vi "Read Matlab Params.vi"(8 "error in (no error)":errorcluster, 10 "Enum":T1(ring), 11 "TrialBasedExperiment in":refnum<class "MatlabExperiment.lvclass">) -> (0 "error out":errorcluster, 2 "Matlab Param Array":cluster{"Name":string, "Data":variant}[](array[cluster]), 3 "TrialBasedExperiment out":refnum<class "MatlabExperiment.lvclass">)   [LabVIEW 2010, in "MatlabExperiment.lvclass"]
uses:
  MatlabExperiment.lvclass
  Matlab API/Matlab API.lvlib
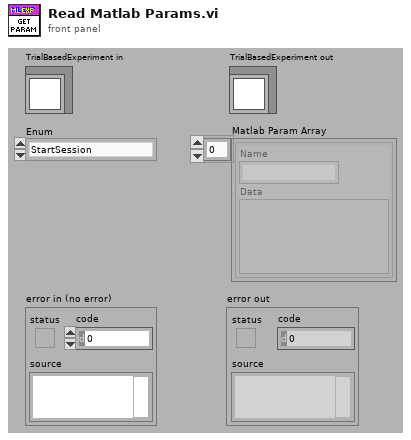
[diagram p1: front panel]
types:
  T1 = enum16{"StartSession", "StartTrial", "ShowStimulus"}
  T2 = cluster{"Name":string, "Type":string, "value":string}[]
  T3 = cluster{"Intertrial":dbl, "AcquireFixation":dbl, "HoldFixation":dbl, "DelayPeriod":dbl, "ResponsePeriod":dbl}
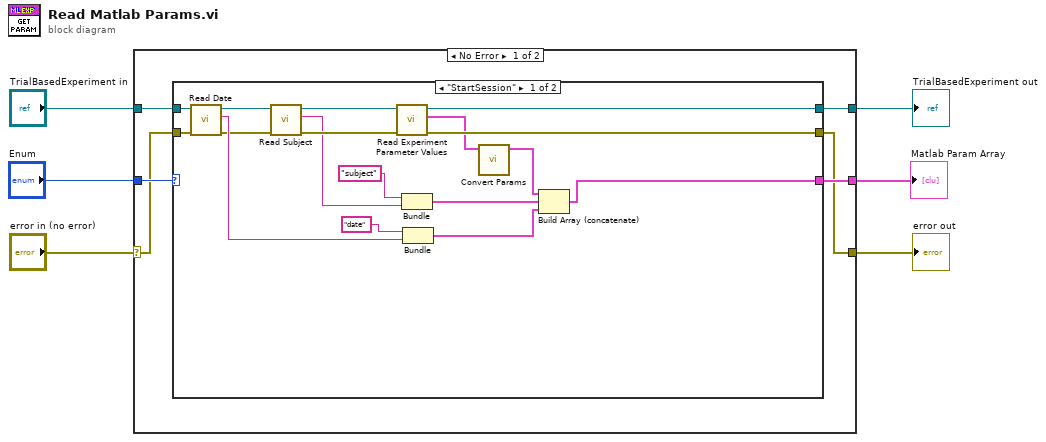
[diagram p0: block diagram]
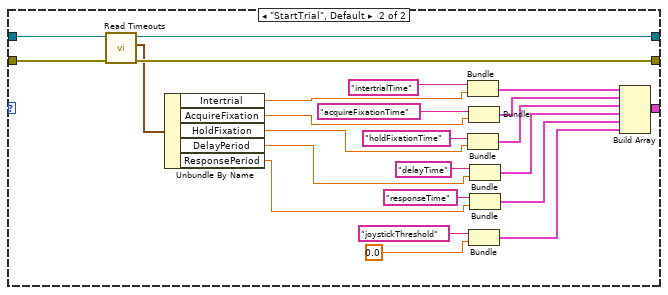
[diagram p2: hidden frame]
diagram:
  n1 = case shown="No Error" "error in (no error)" {
    selector: "error in (no error)" -> [w8 w55]
    tunnel: [w7 w55] -> w5
    tunnel: [w11 w54] -> w3
    tunnel: "TrialBasedExperiment in" -> [w10 w54]
    tunnel: "Enum" -> [w12 _]
    tunnel: [w9 _] -> w1
    frame No Error {
      n2 = case shown="\"StartSession\"" w12 {
        tunnel: [w29 w35] -> w11
        tunnel: w10 -> [w16 w31]
        tunnel: [w20 w32] -> w9
        tunnel: w8 -> [w14 w30]
        tunnel: [w28 w36] -> w7
        frame "StartSession" {
          n3 = call-dynamic "Read Date.vi"("error in (no error)"=w14, "TrialBasedExperiment in"=w16) -> ("error out"=w13:errorcluster, "Date"=w17:string, "TrialBasedExperiment out"=w15:refnum<class "MatlabExperiment.lvclass">)  [unwired: 7 in]
          n4 = call-dynamic "Read Subject.vi"("error in (no error)"=w13, "TrialBasedExperiment in"=w15) -> ("error out"=w27:errorcluster, "Subject"=w24:string, "TrialBasedExperiment out"=w26:refnum<class "MatlabExperiment.lvclass">)  [unwired: 7 in]
          n5 = call-dynamic "Read Experiment Parameter Values.vi"("error in (no error)"=w27, "TrialBasedExperiment in"=w26) -> ("error out"=w28:errorcluster, "Experiment Parameter Values"=w23:T2, "TrialBasedExperiment out"=w29:refnum<class "MatlabExperiment.lvclass">)  [unwired: 7 in]
          n6 = Bundle("subject", "Subject"=w24) -> (w22:cluster{string, "Subject":string})  [unwired: 1 in]
          n7 = Bundle("date", "Date"=w17) -> (w18:cluster{string, "Date":string})  [unwired: 1 in]
          n8 = call "Convert Params.vi"("Experiment Parameter Values"=w23) -> ("Matlab Param Array"=w21:cluster{"Name":string, "Data":variant}[])  [unwired: 10 in]
          n9 = Build Array (concatenate)(w21, w22, w18) -> (w20:cluster{"Name":string, "Data":variant}[])
        }
        frame "StartTrial", Default {
          n10 = call-dynamic "Read Timeouts.vi"("error in (no error)"=w30, "TrialBasedExperiment in"=w31) -> ("error out"=w36:errorcluster, "Timeouts"=w34:T3, "TrialBasedExperiment out"=w35:refnum<class "MatlabExperiment.lvclass">)  [unwired: 7 in]
          n11 = Unbundle By Name(w34) -> ("Intertrial"=w45:dbl, "AcquireFixation"=w44:dbl, "HoldFixation"=w43:dbl, "DelayPeriod"=w42:dbl, "ResponsePeriod"=w41:dbl)
          n12 = Bundle("intertrialTime", "Intertrial"=w45) -> (w49:cluster{string, "Intertrial":dbl})  [unwired: 1 out]
          n13 = Bundle("holdFixationTime", "HoldFixation"=w43) -> (w47:cluster{string, "HoldFixation":dbl})  [unwired: 1 out]
          n14 = Bundle("acquireFixationTime", "AcquireFixation"=w44) -> (w48:cluster{string, "AcquireFixation":dbl})  [unwired: 1 out]
          n15 = Bundle("joystickThreshold", 0.0) -> (w33:cluster{string, dbl})  [unwired: 1 out]
          n16 = Bundle("delayTime", "DelayPeriod"=w42) -> (w40:cluster{string, "DelayPeriod":dbl})  [unwired: 1 out]
          n17 = Bundle("responseTime", "ResponsePeriod"=w41) -> (w39:cluster{string, "ResponsePeriod":dbl})  [unwired: 1 out]
          n18 = Build Array(w49, w48, w47, w40, w39, w33) -> (w32:cluster{string, "ResponsePeriod":dbl}[])
        }
      }
    }
    frame Error {
    }
  }
  "error out" <- w5
  "TrialBasedExperiment out" <- w3
  "Matlab Param Array" <- w1
